vi "Disable_Relays.vi"(8 "error in (no error)":errorcluster caption="entrée d'erreur (pas d'erreur)", 11 "Class Relay_Board 16_Relay_CH340 en entrée":refnum<class "Class Relay_Board 16_Relay_Acer_Micro.lvclass">) -> (0 "error out":errorcluster caption="sortie d'erreur", 3 "Class Relay_Board 16_Relay_CH340 en sortie":refnum<class "Class Relay_Board 16_Relay_Acer_Micro.lvclass">)   [LabVIEW 2020, in "Library Instrument & Equipement.lvlib" / "Library Relay_Board.lvlib" / "Class Relay_Board 16_Relay_Acer_Micro.lvclass"]
uses:
  Class Relay_Board 16_Relay_Acer_Micro.lvclass
  C:/Users/ngarcin/OneDrive - Altyor/Standard TB/Class/Relay_Board/Relay_Board (Default)/Class Relay_Board (Default).lvclass
  Class Relay_Board 16_Relay_Acer_Micro.lvclass/Class Relay_Board 16_Relay_Acer_Micro.ctl
  Commun VI/TypeDef/Liste Error.ctl
  Commun VI/Library Commun.lvlib
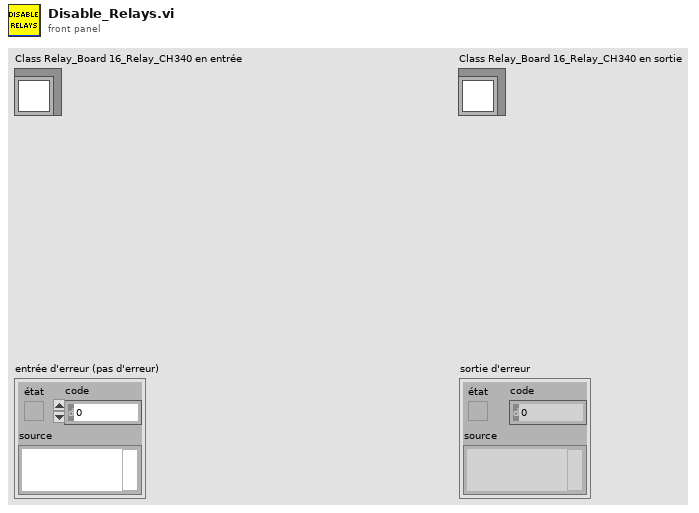
[diagram p1: front panel]
types:
  T1 = typedef "Library Commun.lvlib/Liste Error.ctl" = enum16{"Firebase Driver - Get Document", "Firebase Driver - Get Document With Where", "Firebase Driver - Delete Document", "Firebase Driver - Set Document", "Firebase Driver - Update Document", "Firebase Altyor - Search Document Bench", "Firebase Altyor - Class Not in Firebase", "Spectrum_Analyser - Timeout", "Relay Board - Qty Relay", "DIO - Pb Funtion", "Power_Supply - Peripherical not find", "Mutimeter - Peripherical not find", "Instrument - Function Not Used", "Instrument - Instrument name not specified", "Instrument - Allready Initialised", "Instrument - TimeOut", "Instrument - the instrument must be Initialise before", "Instrument - Frame Not received", "Instrument - Frame Nok", "Test - Initialise the File_for_Save", "Test - Timeout", "Test - Cmd Error", "FGV - Variable ", "BDD FireBase - Define Class", "SN - Class Not Define"}
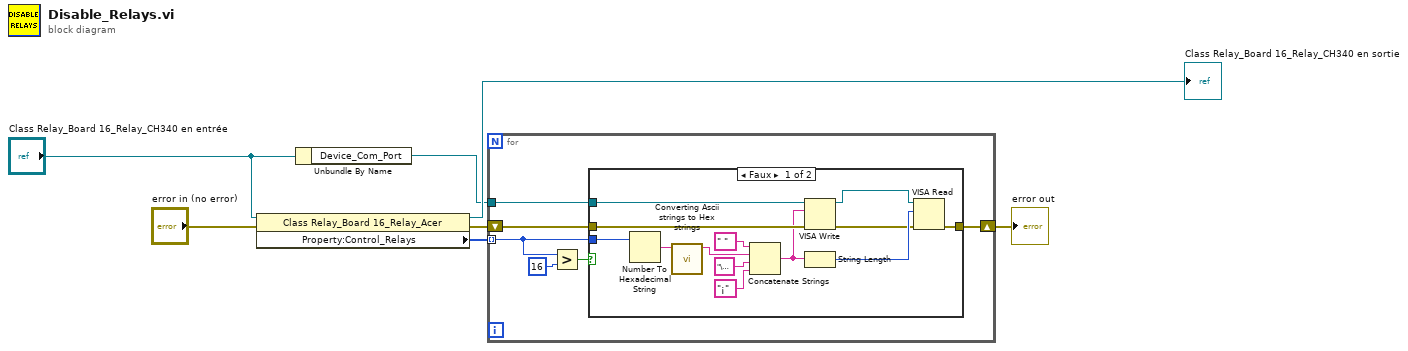
[diagram p0: block diagram]
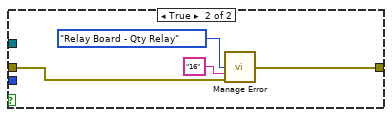
[diagram p2: hidden frame]
diagram:
  n1 = property class="Class Relay_Board 16_Relay_Acer"(reference="Class Relay_Board 16_Relay_CH340 en entrée", error in="error in (no error)") -> (reference out=→"Class Relay_Board 16_Relay_CH340 en sortie":refnum<class "Class Relay_Board 16_Relay_Acer_Micro.lvclass">, error out=w4:errorcluster, "Property:Control_Relays"=w3:u8[])
  n2 = Unbundle By Name("Class Relay_Board 16_Relay_CH340 en entrée") -> ("Device_Com_Port"=w1:refnum<visa-resource-name>)
  n3 = for {
    shift-right: [w11] -> w7
    shift-left: w4 -> [w13]
    tunnel: w3 -> [w9] mode=indexing
    tunnel: w1 -> [w12]
    n4 = Greater?(x=w9, y=u8 16) -> (0:w8:bool)
    n5 = case shown="Faux" w8 {
      tunnel: w13 -> [w24 w27]
      tunnel: w12 -> [w23 _]
      tunnel: w9 -> [w22 _]
      tunnel: [w16 w28] -> w11
      frame False {
        n6 = Number To Hexadecimal String(2:w22) -> (0:w21:string)  [unwired: 1 in]
        n7 = call "Converting Ascii strings to Hex strings.vi"("result string"=w21) -> ("Chaîne"=w20:string)  [unwired: 10 in]
        n8 = Concatenate Strings(" " ("chaîne"), w20, "\u0000" ("chaîne"), "¡" ("chaîne")) -> (w18:string)
        n9 = VISA Write(VISA resource name=w23, write buffer=w18, error in (no error)=w24) -> (VISA resource name out=w17:refnum<visa-resource-name>, error out=w14:errorcluster)  [unwired: 1 out]
        n10 = String Length(string=w18) -> (length=w15:i32)
        n11 = VISA Read(VISA resource name=w17, byte count=w15, error in (no error)=w14) -> (error out=w16:errorcluster)  [unwired: 3 out]
      }
      frame True {
        n12 = call "Manage Error.vi"("Code Erreur"=Liste_Error."Relay Board - Qty Relay", "Text"="16", "error in (no error)"=w27) -> ("error out"=w28:errorcluster)  [unwired: 12 in]
      }
    }
  }
  "error out" <- w7
